vi "absolute.set.vi"(8 "error in (no error)":errorcluster, 10 "absoloute type":refnum<class "ts.absoloute type.lvclass">, 11 "ts.absoloute in":refnum<class "ts.absoloute.lvclass">) -> (0 "error out":errorcluster, 3 "ts.absoloute out":refnum<class "ts.absoloute.lvclass">)   [LabVIEW 2020, in "ts.absoloute.lvclass"]
uses:
  ts.absoloute.lvclass
  ts.absoloute.lvclass/ts.absoloute.ctl
  ts.absoloute type/ts.absoloute type.lvclass
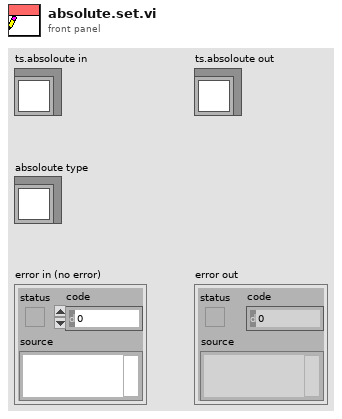
[diagram p1: front panel]
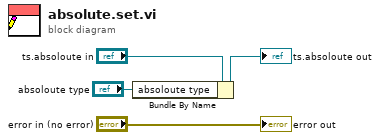
[diagram p0: block diagram]
diagram:
  n1 = Bundle By Name(cluster="ts.absoloute in", "absoloute type"="absoloute type") -> (→"ts.absoloute out":refnum<class "ts.absoloute.lvclass">)
  "error out" <- "error in (no error)"
